vi "MSFET208_pH_CalibCalc.vi"(1 "Eint":dbl=0.9561451648556742) -> (0 "pHint":dbl=6.800997002624105)   [LabVIEW 2018]
panel:
  in  "calpH":dbl=7.0
  in  "calEint":dbl=0.9565
  # "pH Calibration & Calculation (MSFET 208)"
  # "INPUTS"
  # "<-- Automatically inputed"
  # "OUTPUT"
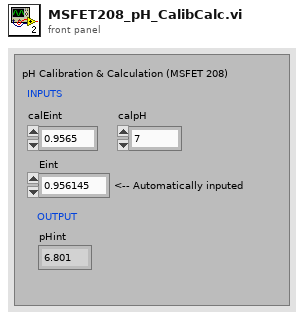
[diagram p1: front panel]
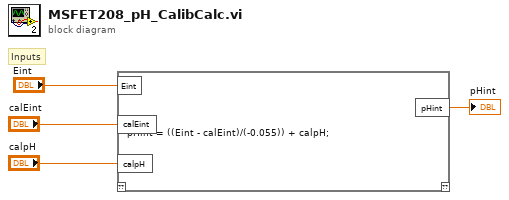
[diagram p0: block diagram]
diagram:
  # "Inputs"
  n1 = script code="pHint = ((Eint - calEint)/(-0.055)) + calpH;"("calEint"="calEint", "calpH"="calpH", "Eint"="Eint") -> ("pHint"=→"pHint":dbl)  [unwired: 1 in, 1 out]
